vi "Write File.vi"(8 "error in":errorcluster, 10 "Data In":refnum<class "Data.lvclass">, 11 "File Obs in":refnum<class "File Observer.lvclass">) -> (0 "error out":errorcluster, 3 "File Obs out":refnum<class "File Observer.lvclass">)   [LabVIEW 2015, in "File Observer.lvclass"]
doc: "Write data to the file specified in File Ref. The default behavior of this VI is to simply write the Data class to a binary file. This VI may be overriden to provide custom functionality."
uses:
  File Observer.lvclass
  Data/Data.lvclass
  File Observer.lvclass/File Observer.ctl
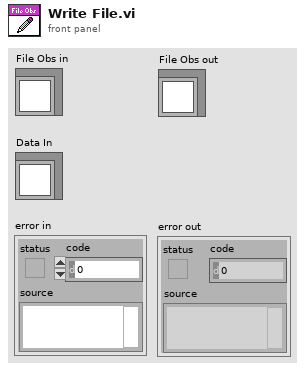
[diagram p1: front panel]
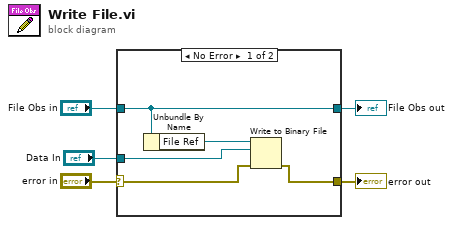
[diagram p0: block diagram]
diagram:
  n1 = case shown="No Error" "error in" {
    selector: "error in" -> [w7 w12]
    tunnel: [w6 w12] -> w4
    tunnel: [w9 w11] -> w2
    tunnel: "File Obs in" -> [w9 w11]
    tunnel: "Data In" -> [w10 _]
    frame No Error {
      n2 = Unbundle By Name(w9) -> ("File Ref"=w8:refnum<file>)
      n3 = Write to Binary File(file (use dialog)=w8, data=w10, error in=w7) -> (error out=w6:errorcluster)  [unwired: 3 in, 2 out]
    }
    frame Error {
    }
  }
  "error out" <- w4
  "File Obs out" <- w2
